vi "Initialize.vi"(8 "error in":errorcluster, 10 "parameters":variant, 11 "node in":refnum<class "WaveformAcq editor node.lvclass">) -> (0 "error out":errorcluster, 2 "summary":T2[](array[typedef]), 3 "data value reference":T1)   [LabVIEW 2017, in "WaveformAcq editor node.lvclass"]
doc: "Initializes the data of a node to its default state.\nThe object is not created inside of this VI, because it is created from a File depending on user selection."
uses:
  WaveformAcq editor node.lvclass
  C:/Program Files (x86)/National Instruments/LabVIEW 2017/vi.lib/NI/Configuration Framework/Node/NISE_CEF_Node.lvclass
  <vilib>/NI/Configuration Framework/Node/Summary.ctl
  <vilib>/NI/Configuration Framework/Node/NodeRef.ctl
  <vilib>/NI/Configuration Framework/Node/NISE_CEF_Node.lvclass
  module/configuration/WaveformAcq configuration.lvclass
  C:/Program Files (x86)/National Instruments/LabVIEW 2017/vi.lib/NI/Configuration Framework/serializable configuration/NISE_CEF_serializable configuration.lvclass
  <vilib>/NI/DCAF/Tag Editor Core/control module/editor node/control module editor.lvclass
  <vilib>/NI/Configuration Framework/serializable configuration/NISE_CEF_serializable configuration.lvclass
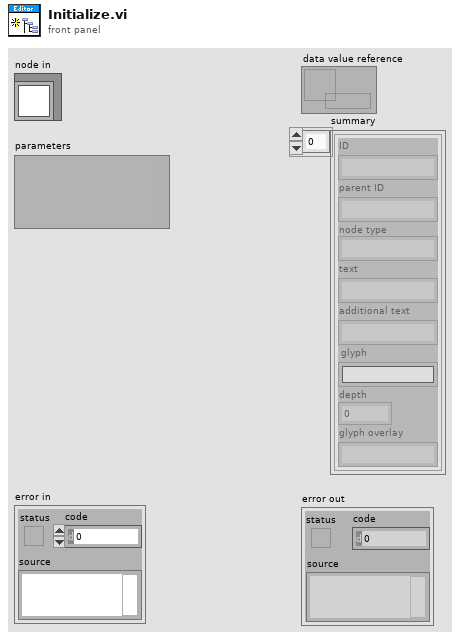
[diagram p1: front panel]
types:
  T1 = typedef "NISE_CEF_Node.lvclass/NodeRef.ctl" = refnum<data-value>
  T2 = typedef "NISE_CEF_Node.lvclass/Summary.ctl" = cluster{"ID":string, "parent ID":string, "node type":string, "text":string, "additional text":string, "glyph":string, "depth":i32, "glyph overlay":string}
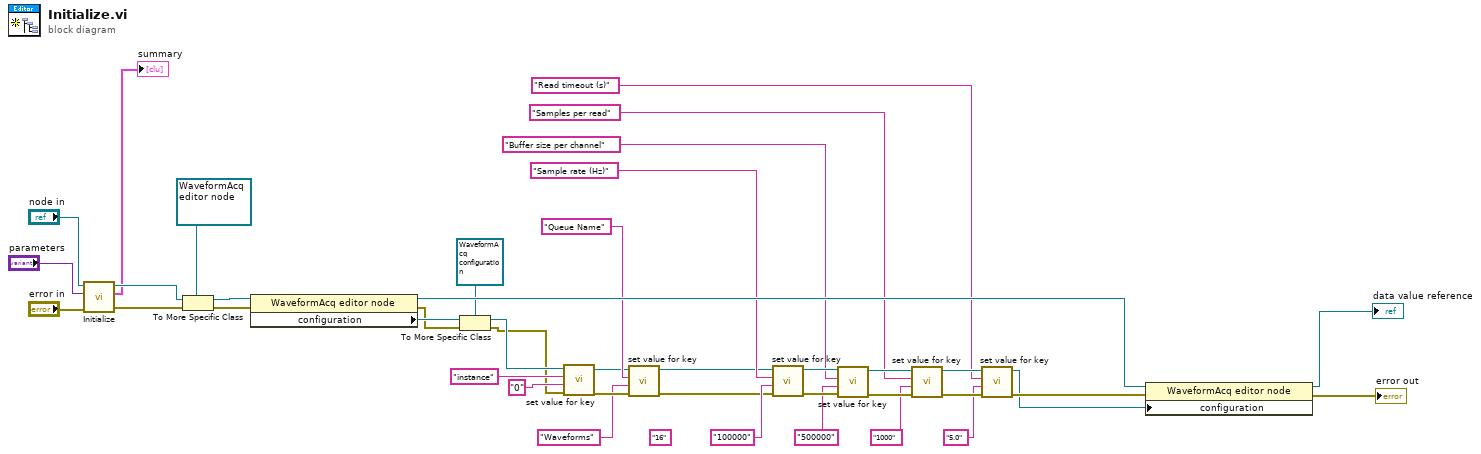
[diagram p0: block diagram]
diagram:
  (unwired) "16" ("value")
  n1 = call-parent "Initialize.vi"("error in"="error in", "parameters"="parameters", "node in"="node in") -> ("error out"=w31:errorcluster, "summary"=→"summary":T2[], "data value reference"=w30:T1)  [unwired: 6 in]
  n2 = To More Specific Class(target class=refnum<data-value> refnum ("data value reference"), reference=w30, error in=w31) -> (specific class reference=w35:refnum<data-value>, error out=w36:errorcluster)
  n3 = property class="WaveformAcq editor node"(reference=w35, error in=w36) -> (reference out=w32:refnum<data-value>, error out=w24:errorcluster, "configuration"=w33:refnum<class "NISE_CEF_serializable configuration.lvclass">)
  n4 = To More Specific Class(target class=refnum<class "WaveformAcq configuration.lvclass"> refnum ("WaveformAcq configuration"), reference=w33, error in=w24) -> (specific class reference=w34:refnum<class "WaveformAcq configuration.lvclass">, error out=w23:errorcluster)
  n5 = call-dynamic "set value for key.vi"("error in"=w23, "value"="0", "key"="instance", "fixed channel configuration in"=w34) -> ("error out"=w20:errorcluster, "fixed channel configuration out"=w21:refnum<class "WaveformAcq configuration.lvclass">)  [unwired: 6 in]
  n6 = call-dynamic "set value for key.vi"("error in"=w20, "value"="Waveforms", "key"="Queue Name" ("String"), "fixed channel configuration in"=w21) -> ("error out"=w2:errorcluster, "fixed channel configuration out"=w1:refnum<class "WaveformAcq configuration.lvclass">)  [unwired: 6 in]
  n7 = call-dynamic "set value for key.vi"("error in"=w2, "value"="100000", "key"="Sample rate (Hz)" ("String"), "fixed channel configuration in"=w1) -> ("error out"=w12:errorcluster, "fixed channel configuration out"=w18:refnum<class "WaveformAcq configuration.lvclass">)  [unwired: 6 in]
  n8 = call-dynamic "set value for key.vi"("error in"=w12, "value"="500000", "key"="Buffer size per channel" ("String"), "fixed channel configuration in"=w18) -> ("error out"=w11:errorcluster, "fixed channel configuration out"=w16:refnum<class "WaveformAcq configuration.lvclass">)  [unwired: 6 in]
  n9 = call-dynamic "set value for key.vi"("error in"=w11, "value"="1000", "key"="Samples per read" ("String"), "fixed channel configuration in"=w16) -> ("error out"=w10:errorcluster, "fixed channel configuration out"=w14:refnum<class "WaveformAcq configuration.lvclass">)  [unwired: 6 in]
  n10 = call-dynamic "set value for key.vi"("error in"=w10, "value"="5.0", "key"="Read timeout (s)" ("String"), "fixed channel configuration in"=w14) -> ("error out"=w9:errorcluster, "fixed channel configuration out"=w8:refnum<class "WaveformAcq configuration.lvclass">)  [unwired: 6 in]
  n11 = property class="WaveformAcq editor node"(reference=w32, error in=w9, "configuration"=w8) -> (reference out=→"data value reference":refnum<data-value>, error out=→"error out":errorcluster)
